vi "ChannelList.vi"   [LabVIEW 2018, in "OXYGEN.lvlib"]
uses:
  OXYGEN.lvlib
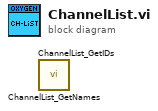
[diagram p0: block diagram]
diagram:
  n1 = call "ChannelList_GetNames.vi"() -> ()  [unwired: 8 in, 4 out]
  n2 = call "ChannelList_GetIDs.vi"() -> ()  [unwired: 8 in, 4 out]
